vi "Calibrate.vi"(8 "error in (no error)":errorcluster, 11 "3446X in":refnum<class "3446X.lvclass">) -> (0 "error out":errorcluster, 1 "Cal Message":string, 2 "Cal Result (Pass=T)":bool, 3 "3446X out":refnum<class "3446X.lvclass">)   [LabVIEW 2018, in "3446X.lvlib" / "3446X.lvclass"]
uses:
  3446X.lvclass
  3446X.lvclass/3446X.ctl
  <instrlib>/Agilent 3446X Series/Agilent 3446X Series.lvlib
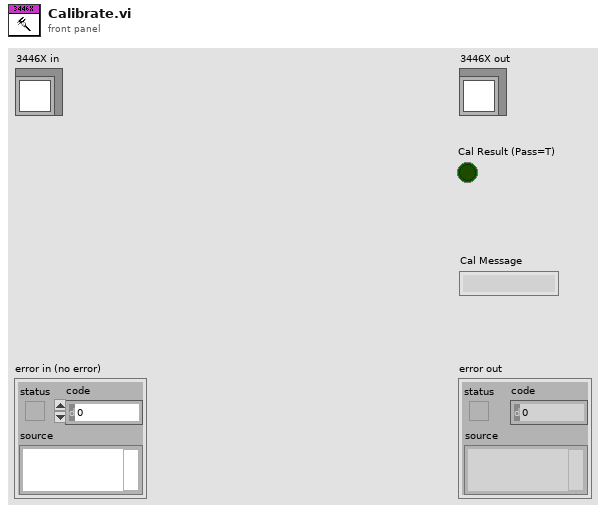
[diagram p1: front panel]
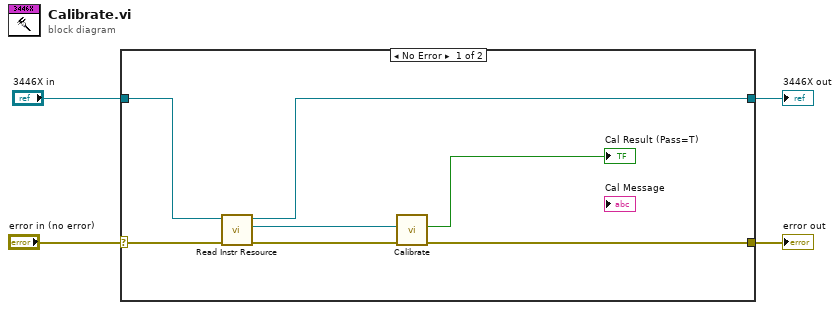
[diagram p0: block diagram]
diagram:
  n1 = case shown="No Error" "error in (no error)" {
    selector: "error in (no error)" -> [w11 w12]
    tunnel: [w7 w13] -> w3
    tunnel: "3446X in" -> [w10 w13]
    tunnel: [w5 w12] -> w1
    frame No Error {
      n2 = call "Read Instr Resource.vi"("error in (no error)"=w11, "3446X in"=w10) -> ("error out"=w9:errorcluster, "Instr Resource"=w8:refnum<visa-resource-name>, "3446X out"=w7:refnum<class "3446X.lvclass">)  [unwired: 7 in]
      n3 = call <instrlib>:"Calibrate.vi"("error in (no error)"=w9, "VISA resource name"=w8) -> ("error out"=w5:errorcluster, "Calibration Result"=→"Cal Result (Pass=T)":bool)  [unwired: 7 in, 1 out]
    }
    frame Error {
    }
  }
  "error out" <- w1
  "3446X out" <- w3
